vi "Is Alarm Clear.vi"(11 "Alarm":T1) -> (3 "Cleared?":bool)   [LabVIEW 2018, in "Dynamic Shared Variables.lvlib"]
uses:
  Dynamic Shared Variables.lvlib
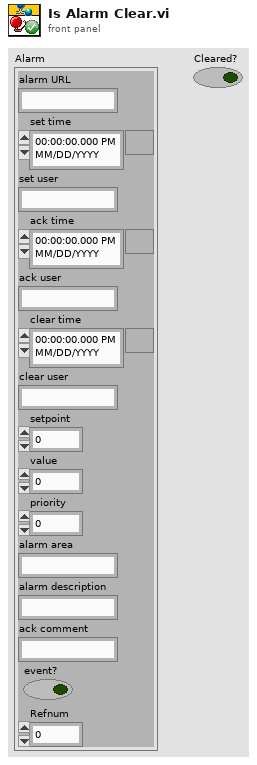
[diagram p1: front panel]
types:
  T1 = cluster{"alarm URL":string, "set time":timestamp, "set user":string, "ack time":timestamp, "ack user":string, "clear time":timestamp, "clear user":string, "setpoint":dbl, "value":dbl, "priority":u32, "alarm area":string, "alarm description":string, "ack comment":string, "event?":bool, "Refnum":u64}
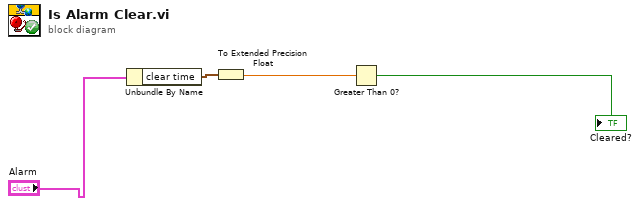
[diagram p0: block diagram]
diagram:
  n1 = Unbundle By Name("Alarm") -> ("clear time"=w4:timestamp)
  n2 = To Extended Precision Float(1:w4) -> (0:w1:ext)
  n3 = Greater Than 0?(x=w1) -> (x > 0?=→"Cleared?":bool)
